vi "ParseSysexCapabilityResponse.vi"(8 "error in":errorcluster={"status"=FALSE, "code"=1073676294, "source"="VISA Read in SerialCommunication.Transport.vi->TransportWrapper.vi->Capability Query.vi->Example.api.vi"}, 10 "Sysex Message":u8[](array[numeric])=[240, 108, 127, 127, 0, 1, 11, 1, 1, 1, 4, 14, 127, 0, 1, 11, 1, 1, 1, 3, 8, 4, 14, 127, 0, 1, 11, 1, 1, 1, 4, 14, 127, 0, 1, 11, 1, 1, 1, 3, 8, 4, 14, 127, 0, 1, 11, 1, 1, 1, 3, 8, 4, 14, 127, 0, 1, 11, 1, 1, 1, 4, 14, 127, 0, 1, 11, 1, 1, 1, 4, 14, 127, 0, 1, 11, 1, 1, 1, 3, 8, 4, 14, 127, 0, 1, 11, 1, 1, 1, 3, 8, 4, 14, 127, 0, 1, 11, 1, 1, 1, 3, 8, 4, 14, 127, 0, 1, 11, 1, 1, 1, 4, 14, 127, 0, 1, 11, 1, 1, 1, 4, 14, 127, 0, 1, 11, 1, 1, 1, 2, 10, 4, 14, 127, 0, 1, 11, 1, 1, 1, 2, 10, 4, 14, 127, 0, 1, 11, 1, 1, 1, 2, 10, 4, 14, 127, 0, 1, 11, 1, 1, 1, 2, 10, 4, 14, 127, 0, 1, 11, 1, 1, 1, 2, 10, 4, 14, 6, 1, 127, 0, 1, 11, 1, 1, 1, 2, 10, 4, 14, 6, 1, 127, 247] format="%x") -> (0 "error out":errorcluster={"status"=FALSE, "code"=1073676294, "source"="VISA Read in SerialCommunication.Transport.vi->TransportWrapper.vi->Capability Query.vi->Example.api.vi"}, 1 "IsValidSysex":bool=TRUE, 2 "Map":map{i32, T1}(c390))   [LabVIEW 2020, in "FirmataClient.lvlib"]
doc: "Parse a message according to the Firmata Protocol Requirements. \n- https://github.com/firmata/protocol\n- https://github.com/firmata/protocol/blob/master/protocol.md"
uses:
  Controls/FirmataPinCapabilitiesAndAnalogMapping.ctl
  Controls/FirmataPinCapability.ctl
  Controls/FirmataPinModes.ctl
  Controls/FirmataProtocolConstants.ctl
  FirmataClient.lvlib
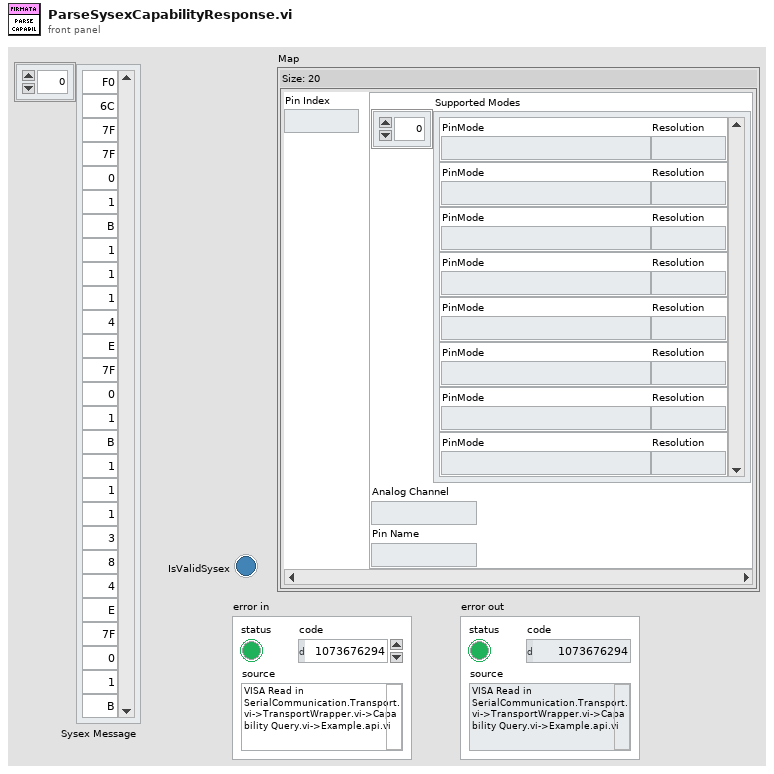
[diagram p1: front panel]
types:
  T1 = typedef "FirmataClient.lvlib/FirmataPinCapabilitiesAndAnalogMapping.ctl" = cluster{"Supported Modes":T2[], "Analog Channel":u8, "Pin Name":string}
  T2 = typedef "FirmataClient.lvlib/FirmataPinCapability.ctl" = cluster{"PinMode":T3, "Resolution":u8}
  T3 = typedef "FirmataClient.lvlib/FirmataPinModes.ctl" = enum16{"DigitalInput", "DigitalOutput", "AnalogInput", "PWM", "Servo", "Shift", "I2C", "OneWire", "Stepper", "Encoder", "Serial", "InputPullup", "Extended.SPI", "Extended.Sonar", "Extended.Tone", "Extended.DHT"}
  T4 = typedef "FirmataClient.lvlib/FirmataProtocolConstants.ctl" = u16
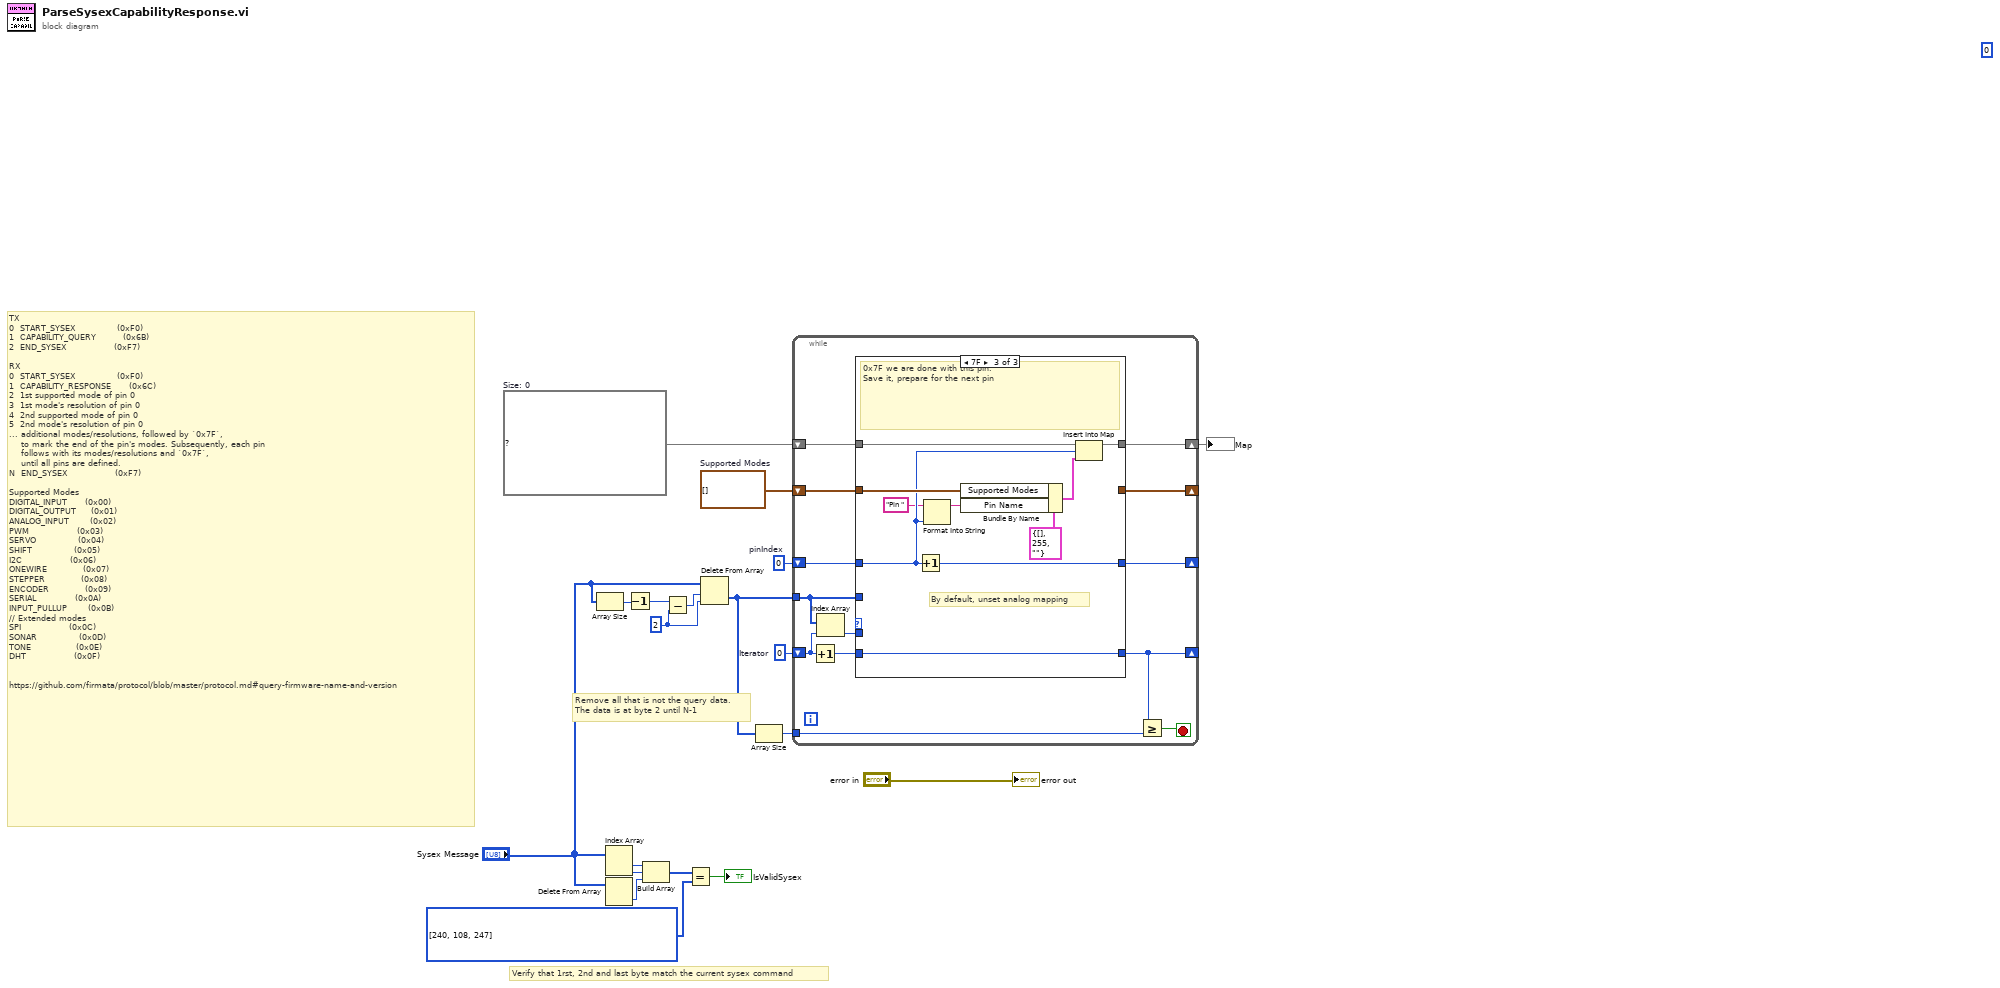
[diagram p0: block diagram]
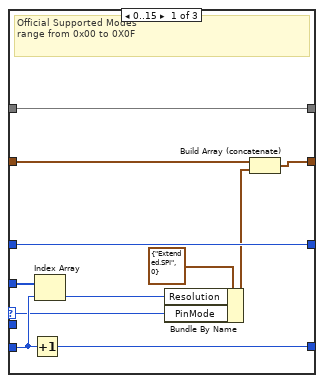
[diagram p2: hidden frame]
diagram:
  w3 = T2[] []  # Supported Modes
  (unwired) 0
  w4 = map{i32, T1} {}  # Size: 0
  w5 = 0  # pinIndex
  w6 = T4[] [240, 108, 247] items=["ANALOG_IO_MESSAGE"=224, "DIGITAL_IO_MESSAGE"=144, "REPORT_ANALOG_PIN"=192, "REPORT_DIGITAL_PORT"=208, "START_SYSEX"=240, "END_SYSEX"=247, "SET_PIN_MODE"=244, "SET_DIGITAL_PIN_VALUE"=245, "PROTOCOL_VERSION"=249, "SYSTEM_RESET"=255, "SYSEX.EXTENDED_ID"=0, "SYSEX.RESERVED_USER_COMMANDs"=1, "SYSEX.ANALOG_MAPPING_QUERY"=105, "SYSEX.ANALOG_MAPPING_RESPONSE"=106, "SYSEX.CAPABILITY_QUERY"=107, "SYSEX.CAPABILITY_RESPONSE"=108, "SYSEX.PIN_STATE_QUERY"=109, "SYSEX.PIN_STATE_RESPONSE"=110, "SYSEX.REPORT_FIRMWARE"=121, "SYSEX.EXTENDED_ANALOG"=111, "SYSEX.STRING_DATA"=113, "SYSEX.REALTIME"=127, "SYSEX.NON_REALTIME"=126, "SYSEX.SAMPLING_INTERVAL"=122, "FEATURES.SYSEX.I2C_READ_WRITE"=118, "FEATURES.SYSEX.I2C_REPLY"=119, "FEATURES.SYSEX.I2C_CONFIG"=120]
  w9 = 0  # Iterator
  w12 = 2 ("index")
  # "Remove all that is not the query data. \nThe data is at byte 2 until N-1"
  # "Verify that 1rst, 2nd and last byte match the current sysex command"
  # "TX\n0  START_SYSEX              (0xF0)\n1  CAPABILITY_QUERY         (0x6B)\n2  END_SYSEX                (0xF7)\n\nRX\n0  START_SYSEX              (0xF0)\n1  CAPABILITY_RESPONSE      (0x6C)\n2  1st supported mode of pin 0\n3  1st mode's resolution of pin 0\n4  2nd supported mode of pin 0\n5  2nd mode's resolution of pin 0\n... additional modes/resolutions, followed by `0x7F`,\n    to mark the end of the pin's modes. Subsequently, each pin\n    follows with its modes/resolutions and `0x7F`,\n    until all pins are defined.\nN  END_SYSEX                (0xF7)\n\nSupported Modes\nDIGITAL_INPUT      (0x00)\nDIGITAL_OUTPUT     (0x01)\nANALOG_INPUT       (0x02)\nPWM                (0x03)\nSERVO              (0x04)\nSHIFT              (0x05)\nI2C                (0x06)\nONEWIRE            (0x07)\nSTEPPER            (0x08)\nENCODER            (0x09)\nSERIAL             (0x0A)\nINPUT_PULLUP       (0x0B)\n// Extended modes \nSPI                (0x0C)\nSONAR              (0x0D)\nTONE               (0x0E)\nDHT                (0x0F)\n\n\nhttps://github.com/firmata/protocol/blob/master/protocol.md#query-firmware-name-and-version"
  n1 = Array Size(array="Sysex Message") -> (size(s)=w14:i32)
  n2 = Index Array(array="Sysex Message") -> (element #1=w19:u8, element #2=w17:u8)  [unwired: 2 in]
  n3 = Delete From Array(array="Sysex Message") -> (deleted portion=w18:u8)  [unwired: 2 in, 1 out]
  n4 = Decrement(x=w14) -> (x-1=w13:i32)
  n5 = Build Array(w19, w17, w18) -> (w16:u8[])
  n6 = Subtract(x=w13, y=w12) -> (x-y=w11:i32)
  n7 = Equal?(x=w16, y=w6) -> (x = y?=→"IsValidSysex":bool)
  n8 = Delete From Array(array="Sysex Message", length=w11, index=w12) -> (deleted portion=w8:u8[])  [unwired: 1 out]
  n9 = Array Size(array=w8) -> (size(s)=w7:i32)
  n10 = while {
    tunnel: w8 -> [w30]
    shift-right: [w28] -> _
    shift-left: w9 -> [w32]
    tunnel: w7 -> [w26]
    shift-right: [w24] -> _
    shift-left: w5 -> [w25]
    shift-right: [w23] -> w1
    shift-left: w4 -> [w22]
    shift-right: [w21] -> _
    shift-left: w3 -> [w20]
    stop <- w27 stop-if-true
    n11 = Increment(x=w32) -> (x+1=w31:i32)
    n12 = Index Array(array=w30, index=w32) -> (element=w29:u8)
    n13 = case shown="7F" w29 {
      selector: w29 -> [w33 _ _]
      tunnel: w31 -> [w42 w47 w57]
      tunnel: w30 -> [w43 _ _]
      tunnel: w29 -> [_ _ _]
      tunnel: [w41 w47 w57] -> w28
      tunnel: w25 -> [w39 w46 w49]
      tunnel: [w39 w46 w50] -> w24
      tunnel: [w38 w45 w55] -> w23
      tunnel: w22 -> [w38 w45 w56]
      tunnel: [w36 w44 _] -> w21
      tunnel: w20 -> [w37 w44 w53]
      frame 0..15 {
        # "Official Supported Modes\nrange from 0x00 to 0X0F"
        n14 = Increment(x=w42) -> (x+1=w41:i32)
        n15 = Index Array(array=w43, index=w42) -> (element=w40:u8)
        n16 = Bundle By Name(cluster=T2 {"PinMode"=enum."Extended.SPI", "Resolution"=0}, "Resolution"=w40, "PinMode"=w33) -> (w34:T2)
        n17 = Build Array (concatenate)(w37, w34) -> (w36:T2[])
      }
      frame Default {
      }
      frame 127 {
        # "By default, unset analog mapping"
        # "0x7F we are done with this pin.\nSave it, prepare for the next pin"
        n18 = Increment(x=w49) -> (x+1=w50:i32)
        n19 = Format Into String(initial string="Pin ", w49) -> (resulting string=w51:string)  [unwired: 2 in, 1 out]
        n20 = Bundle By Name(cluster=T1 {"Supported Modes"=[], "Analog Channel"=255, "Pin Name"=""} ("value"), "Supported Modes"=w53, "Pin Name"=w51) -> (w52:T1)
        n21 = Insert Into Map(map in=w56, key=w49, value=w52) -> (map out=w55:map{i32, T1})  [unwired: 2 out]
      }
    }
    n22 = Greater Or Equal?(x=w28, y=w26) -> (x >= y?=w27:bool)
  }
  "Map" <- w1
  "error out" <- "error in"
